vi "Set FFT Config.vi"(8 "error in (no error)":errorcluster, 10 "CPU FFT Size":u64=2000000 format="%.0p Samples", 11 "CPU FFT Calculator in":refnum<class "CPU FFT Calculator.lvclass">) -> (0 "error out":errorcluster, 3 "CPU FFT Calculator out":refnum<class "CPU FFT Calculator.lvclass">)   [LabVIEW 2020, in "CPU FFT Calculator.lvlib" / "CPU FFT Calculator.lvclass"]
uses:
  CPU FFT Calculator.lvclass
  CPU FFT Calculator.lvclass/CPU FFT Calculator.ctl
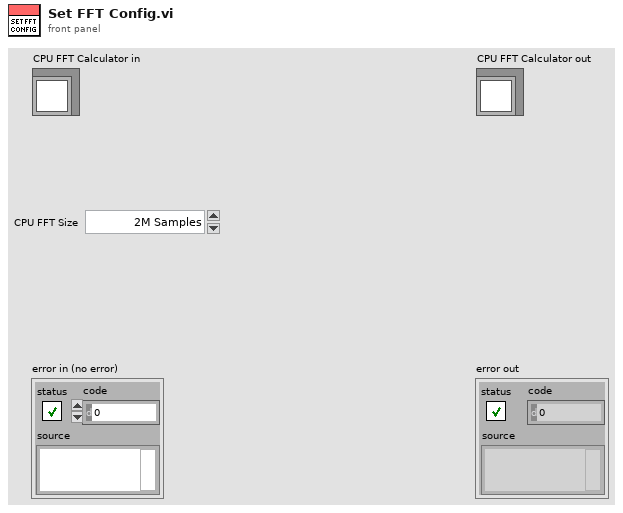
[diagram p1: front panel]
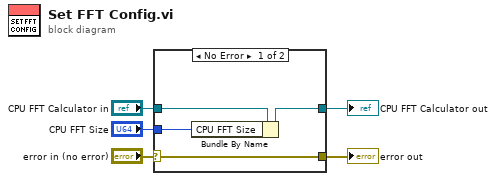
[diagram p0: block diagram]
diagram:
  n1 = case shown="No Error" "error in (no error)" {
    selector: "error in (no error)" -> [w8 w11]
    tunnel: [w8 w11] -> w4
    tunnel: [w7 w10] -> w2
    tunnel: "CPU FFT Calculator in" -> [w9 w10]
    tunnel: "CPU FFT Size" -> [w6 _]
    frame No Error {
      n2 = Bundle By Name(cluster=w9, "CPU FFT Size"=w6) -> (w7:refnum<class "CPU FFT Calculator.lvclass">)
    }
    frame Error {
    }
  }
  "error out" <- w4
  "CPU FFT Calculator out" <- w2
